vi "Do.vi"(8 "error in (no error)":errorcluster, 10 "Actor in":refnum<class "Actor.lvclass">, 11 "Add User Msg":refnum<class "Add User Msg.lvclass">) -> (0 "error out":errorcluster, 2 "Actor out":refnum<class "Actor.lvclass">)   [LabVIEW 2017, in "User Manager Model.lvlib" / "Add User Msg.lvclass"]
doc: "This VI delivers the message to the actor by calling the appropriate method(s) on the actor."
uses:
  <vilib>/gpm_packages/@cs/User Manager App/User Manager Model/User Manager Model Messages/Add User Msg/Add User Msg.lvclass
  <vilib>/ActorFramework/Actor/Actor.lvclass
  <vilib>/gpm_packages/@cs/User Manager App/User Manager Model/User Manager Model/User Manager Model.lvclass
  C:/Program Files/National Instruments/LabVIEW 2017/vi.lib/ActorFramework/Actor/Actor.lvclass
  <vilib>/gpm_packages/@cs/User Manager App/User Manager Model/Type Definitions/New User Information.ctl
  <vilib>/gpm_packages/@cs/User Manager App/User Manager Model/Type Definitions/Credentials.ctl
  <vilib>/gpm_packages/@cs/User Manager App/User Manager Model/Type Definitions/User Levels.ctl
  <vilib>/gpm_packages/@cs/User Manager App/User Manager Model/Type Definitions/User Manager Application Types.lvlib
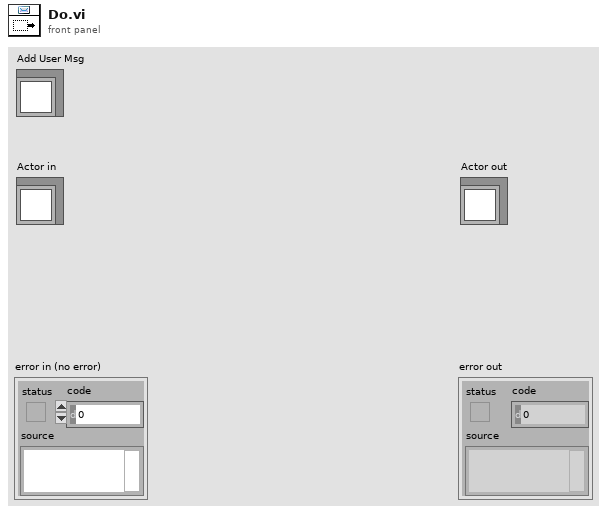
[diagram p1: front panel]
types:
  T1 = typedef "User Manager Application Types.lvlib/New User Information.ctl" = cluster{"User Info":T2, "User Level":T3}
  T2 = typedef "User Manager Application Types.lvlib/Credentials.ctl" = cluster{"Username":string, "Password":string}
  T3 = typedef "User Manager Application Types.lvlib/User Levels.ctl" = cluster{"Rank":i32, "Title":string}
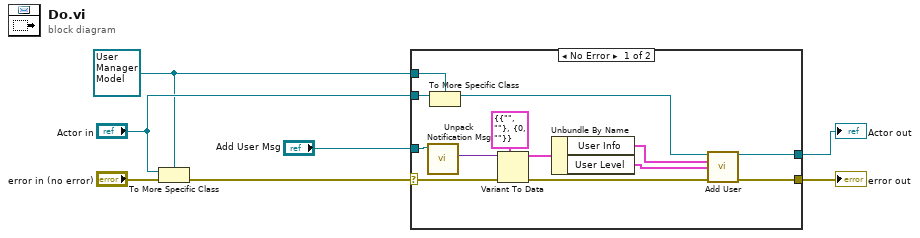
[diagram p0: block diagram]
diagram:
  w2 = refnum<class "User Manager Model.lvclass"> refnum ("Actor in")
  n1 = To More Specific Class(target class=w2, reference="Actor in", error in="error in (no error)") -> (error out=w6:errorcluster)  [unwired: 1 out]
  n2 = case shown="No Error" w6 {
    selector: w6 -> [w13 w22]
    tunnel: [w20 w22] -> w5
    tunnel: [w19 w21] -> w4
    tunnel: "Actor in" -> [w18 w21]
    tunnel: w2 -> [w17 _]
    tunnel: "Add User Msg" -> [w15 _]
    frame No Error {
      n3 = call-dynamic "Unpack Notification Msg.vi"("Notification Msg"=w15) -> ("Value"=w14:variant)  [unwired: 8 in, 2 out]
      n4 = To More Specific Class(target class=w17, reference=w18) -> (specific class reference=w16:refnum<class "User Manager Model.lvclass">)  [unwired: 1 in, 1 out]
      n5 = Variant To Data(error in=w13, type=T1 {"User Info"={"Username"="", "Password"=""}, "User Level"={"Rank"=0, "Title"=""}}, Variant=w14) -> (data=w11:T1, error out=w8:errorcluster)
      n6 = Unbundle By Name(w11) -> ("User Info"=w10:T2, "User Level"=w9:T3)
      n7 = call <vilib>:"Add User.vi"("User Manager Model in"=w16, "User Info"=w10, "User Level"=w9, "error in (no error)"=w8) -> ("User Manager Model out"=w19:refnum<class "User Manager Model.lvclass">, "error out"=w20:errorcluster)  [unwired: 10 in]
    }
    frame Error {
      # "If type check fails, pass the original object out again."
    }
  }
  "error out" <- w5
  "Actor out" <- w4
